vi "Dataflow.vi"() -> ()   [LabVIEW 2010]
doc: "A sample VI used to demonstrate dataflow."
panel:
  out "C":dbl
  in  "B":dbl=3.0 min=0.0 max=100.0 step=1.0
  in  "A":dbl=2.0
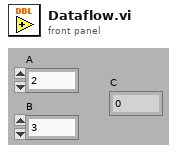
[diagram p1: front panel]
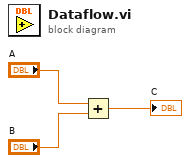
[diagram p0: block diagram]
diagram:
  n1 = Add(x="A", y="B") -> (x+y=→"C":dbl)
